vi "Update Plots.vi"(8 "error in (no error)":errorcluster, 10 "File Path":path, 11 "Application Controller in":refnum<class "Application Controller.lvclass">) -> (0 "error out":errorcluster, 3 "Application Controller out":refnum<class "Application Controller.lvclass">)   [LabVIEW 2018, in "Application Controller.lvclass"]
uses:
  Application Controller.lvclass
  Application Controller.lvclass/Application Controller.ctl
  <vilib>/ActorFramework/Message Enqueuer/Message Enqueuer.lvclass
  Plots/XY Plot Messages/File updated Msg/File updated Msg.lvclass/File updated Msg.ctl
  <vilib>/ActorFramework/Message Enqueuer/Message Enqueuer.lvclass/Message Enqueuer.ctl
  <vilib>/ActorFramework/Message Enqueuer/Enqueue.vi
  Plots/XY Plot Messages/File updated Msg/File updated Msg.lvclass
  C:/Program Files/National Instruments/LabVIEW 2018/vi.lib/ActorFramework/Message/Message.lvclass
  <vilib>/ActorFramework/Message Priority Queue/Priority Enqueue.vi
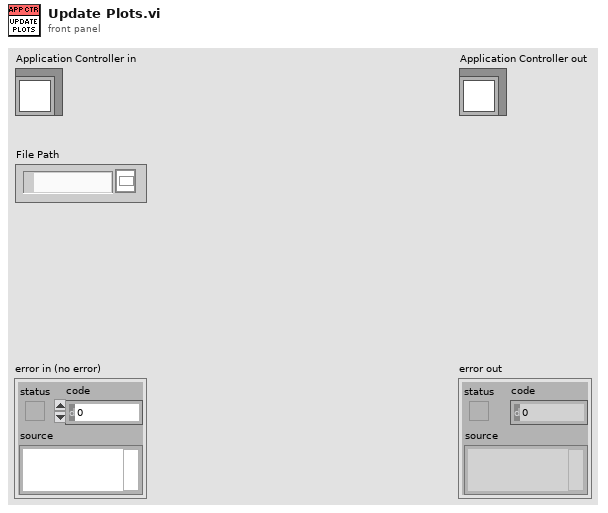
[diagram p1: front panel]
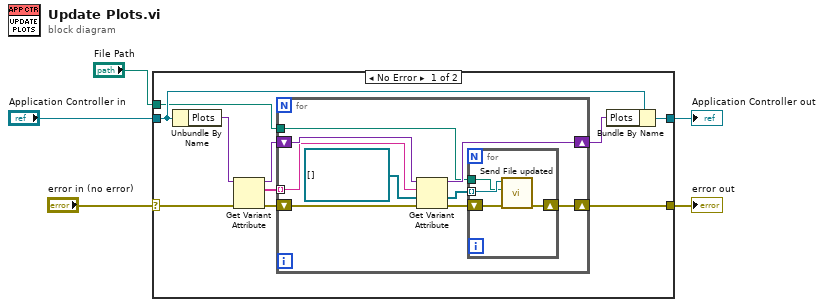
[diagram p0: block diagram]
diagram:
  n1 = case shown="No Error" "error in (no error)" {
    selector: "error in (no error)" -> [w10 w30]
    tunnel: [w9 w30] -> w4
    tunnel: [w8 w29] -> w2
    tunnel: "Application Controller in" -> [w15 w29]
    tunnel: "File Path" -> [w6 _]
    frame No Error {
      n2 = Unbundle By Name(w15) -> ("Plots"=w11:variant)
      n3 = Get Variant Attribute(Variant=w11, error in=w10) -> (duplicate Variant=w13:variant, names=w12:string[], error out=w14:errorcluster)  [unwired: 2 in, 1 out]
      n4 = for {
        tunnel: w12 -> [w21] mode=indexing
        shift-right: [w17] -> w9
        shift-left: w14 -> [w23]
        shift-right: [w20] -> w7
        shift-left: w13 -> [w24]
        tunnel: w6 -> [w16]
        n5 = Get Variant Attribute(Variant=w24, name=w21, default value (empty Variant)=refnum<class "Message Enqueuer.lvclass">[] [] ("Plot enqueuers"), error in=w23) -> (duplicate Variant=w20:variant, value=w19:refnum<class "Message Enqueuer.lvclass">[], error out=w18:errorcluster)  [unwired: 1 out]
        n6 = for {
          tunnel: w19 -> [w28] mode=indexing
          tunnel: w16 -> [w27]
          shift-right: [w25] -> w17
          shift-left: w18 -> [w26]
          n7 = call "Send File updated.vi"("error in (no error)"=w26, "File Path Control"=w27, "Message Enqueuer"=w28) -> ("error out"=w25:errorcluster)  [unwired: 7 in, 1 out]
        }
      }
      n8 = Bundle By Name(cluster=w15, "Plots"=w7) -> (w8:refnum<class "Application Controller.lvclass">)
    }
    frame Error {
    }
  }
  "error out" <- w4
  "Application Controller out" <- w2
